vi "Read FPENs.vi"(3 "FP":refnum<class "DecFrame_FP.lvclass">) -> (1 "FPEN":refnum<class "FPEN.lvclass">)   [LabVIEW 2023, in "DecFrame_FP.lvclass"]
uses:
  DecFrame_FP/DecFrame_FP.lvclass
  FPEN/FPEN.lvclass
  DecFrame_FP/DecFrame_FP.lvclass/DecFrame_FP.ctl
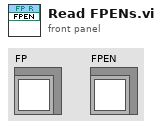
[diagram p1: front panel]
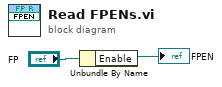
[diagram p0: block diagram]
diagram:
  n1 = Unbundle By Name("FP") -> ("Enable"=→"FPEN":refnum<class "FPEN.lvclass">)
